vi "Read Waveform from TDMS (Unscaled Int8).vi"(0 "VISA resource name":refnum<visa-resource-name>, 1 "Start Point (0)":i32, 2 "TDMS Path":path, 5 "Measurement Source (1: Channel 1)":i32(ring)=1 items=["Channel 1"=1, "Channel 2"=2, "Channel 3"=3, "Channel 4"=4, "Function 1"=5, "Function 2"=6, "Function 3"=7, "Function 4"=8, "Memory 1"=9, "Memory 2"=10, "Memory 3"=11, "Memory 4"=12], 7 "Length (1000)":i32=10000 caption="Length (10000)", 11 "error in (no error)":errorcluster) -> (4 "VISA resource name out":refnum<visa-resource-name>, 6 "Waveform Information":T1, 8 "Waveform Data":i8[](array[numeric]), 15 "error out":errorcluster)   [LabVIEW 2013, in "Agilent 90000 Series.lvlib"]
doc: "Returns a block of Int8 raw data stored in a TDMS file."
uses:
  Agilent 90000 Series.lvlib
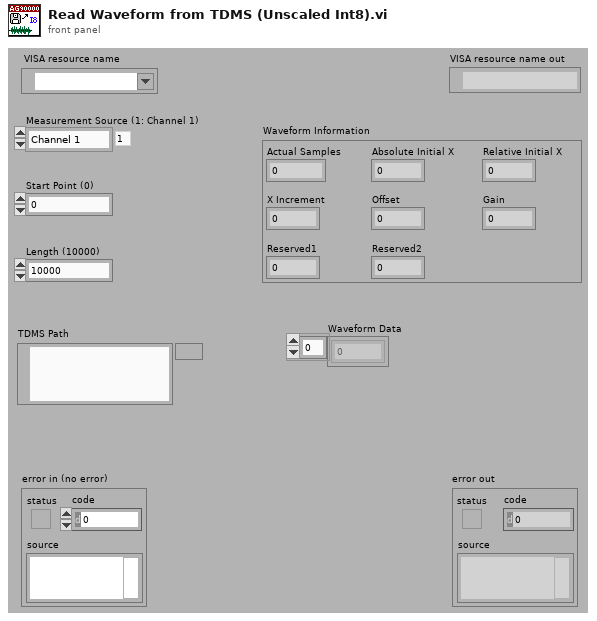
[diagram p1: front panel]
types:
  T1 = cluster{"Actual Samples":i32, "Absolute Initial X":dbl, "Relative Initial X":dbl, "X Increment":dbl, "Offset":dbl, "Gain":dbl, "Reserved1":dbl, "Reserved2":dbl}
  T2 = enum16{"open", "open or create", "create or replace", "create", "open (read-only)"}
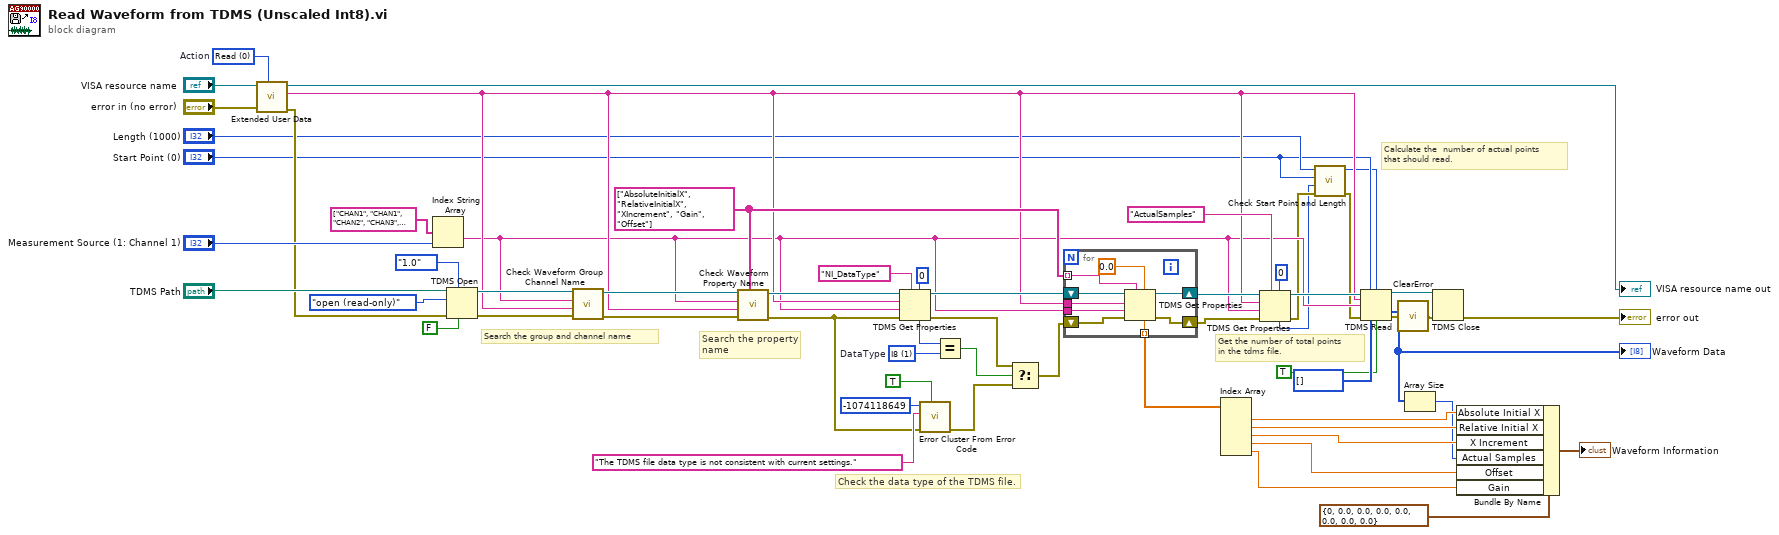
[diagram p0: block diagram]
diagram:
  w21 = u16 0 items=["Read", "Write"]  # Action
  w31 = string[] ["AbsoluteInitialX", "RelativeInitialX", "XIncrement", "Gain", "Offset"] ("property names")
  w52 = u16 1 items=["I8"=1, "I16"=2, "I32"=3, "DBL"=10]  # DataType
  # "Calculate the  number of actual points\nthat should read."
  # "Get the number of total points\nin the tdms file."
  # "Check the data type of the TDMS file."
  # "Search the property\nname"
  # "Search the group and channel name"
  n1 = call "Extended User Data.vi"("Action"=w21, "Error In (no error)"="error in (no error)", "VISA resource name in"="VISA resource name") -> ("Error Out"=w19:errorcluster, "Default Group Name Out"=w13:string, "VISA resource name out"=→"VISA resource name out":refnum<visa-resource-name>)  [unwired: 1 in, 5 out]
  n2 = Index String Array(1:"Measurement Source (1: Channel 1)", 2:string[] ["CHAN1", "CHAN1", "CHAN2", "CHAN3", "CHAN4", "FUNC1", "FUNC2", "FUNC3", "FUNC4", "WMEM1", "WMEM2", "WMEM3", "WMEM4"] ("subarray 2")) -> (0:w12:string)  [unwired: 1 out]
  n3 = TDMS Open(6:FALSE ("disable buffering? (T)"), 7:enum16{"1.0", "2.0"}."1.0" ("file format version (2.0)"), 8:w19, 10:T2."open (read-only)" ("operation (0:open)"), 11:"TDMS Path") -> (0:w29:errorcluster, 3:w30:refnum<k34>)  [unwired: 2 in]
  n4 = call "Check Waveform Group Channel Name.vi"("error in (no error)"=w29, "Group Name"=w13, "Channel Name"=w12, "TDMS File In"=w30) -> ("error out"=w28:errorcluster, "TDMS File Out"=w27:refnum<k34>)  [unwired: 6 out]
  n5 = call "Check Waveform Property Name.vi"("Property Name"=w31, "error in (no error)"=w28, "Group Name"=w13, "Channel Name"=w12, "TDMS File In"=w27) -> ("error out"=w32:errorcluster, "TDMS File Out"=w45:refnum<k34>)  [unwired: 5 out]
  n6 = TDMS Get Properties(5:u16 0 ("Ring"), 7:"NI_DataType" ("property name"), 8:w32, 9:w12, 10:w13, 11:w45) -> (0:w50:errorcluster, 3:w43:refnum<k34>, 4:w53:u16)  [unwired: 3 out]
  n7 = call <vilib>:"Error Cluster From Error Code.vi"("show call chain? (False)"=TRUE, "error in (no error)"=w32, "error message (\"\")"="The TDMS file data type is not consistent with current settings." ("error message (\"\")"), "error code (0)"=-1074118649) -> ("error out"=w46:errorcluster)  [unwired: 5 out]
  n8 = Equal?(x=w53, y=w52) -> (x = y?=w51:bool)
  n9 = Select(t=w50, s=w51, f=w46) -> (s? t:f=w42:errorcluster)
  n10 = for {
    tunnel: w12 -> [w65]
    tunnel: w13 -> [w64]
    shift-right: [w66] -> w17
    shift-left: w42 -> [w67]
    tunnel: w31 -> [w62] mode=indexing
    tunnel: [w60] -> w41 mode=indexing
    shift-right: [w63] -> w15
    shift-left: w43 -> [w68]
    n11 = TDMS Get Properties(5:0.0 ("Reserved1"), 7:w62, 8:w67, 9:w65, 10:w64, 11:w68) -> (0:w66:errorcluster, 3:w63:refnum<k34>, 4:w60:dbl)  [unwired: 3 out]
  }
  n12 = Index Array(array=w41) -> (element #1=w40:dbl, element #2=w39:dbl, element #3=w38:dbl, element #4=w25:dbl, element #5=w24:dbl)  [unwired: 5 in]
  n13 = TDMS Get Properties(5:0 ("Ring"), 7:"ActualSamples" ("property name"), 8:w17, 9:w12, 10:w13, 11:w15) -> (0:w10:errorcluster, 3:w16:refnum<k34>, 4:w8:i32)  [unwired: 3 out]
  n14 = call "Check Start Point and Length.vi"("error in (no error)"=w10, "Total Samples in TDMS (10000)"=w8, "Start Point (0)"="Start Point (0)", "Length (1000)"="Length (1000)") -> ("error out"=w11:errorcluster, "Actual Points"=w6:i32)  [unwired: 6 out]
  n15 = TDMS Read(0:w16, 1:"Start Point (0)", 2:w6, 5:w13, 7:w12, 11:w11, 12:i8[] [], 13:TRUE ("return channels in file order? (F)")) -> (4:w34:refnum<k34>, 10:w5:i8[], 15:w3:errorcluster)  [unwired: 3 out]
  "Waveform Data" <- w5
  n16 = call <vilib>:"ClearError.vi"("error in (no error)"=w3) -> ("error out"=w35:errorcluster)
  n17 = Array Size(array=w5) -> (size(s)=w33:i32)
  n18 = TDMS Close(8:w35, 11:w34) -> (0:→"error out":errorcluster)  [unwired: 1 out]
  n19 = Bundle By Name(cluster=T1 {"Actual Samples"=0, "Absolute Initial X"=0.0, "Relative Initial X"=0.0, "X Increment"=0.0, "Offset"=0.0, "Gain"=0.0, "Reserved1"=0.0, "Reserved2"=0.0} ("Waveform Information"), "Absolute Initial X"=w40, "Relative Initial X"=w39, "X Increment"=w38, "Actual Samples"=w33, "Offset"=w25, "Gain"=w24) -> (→"Waveform Information":T1)
